vi "Simple 48-bit adder.vi"(8 "Input Valid":bool=TRUE, 10 "B":fxp<+/-,48,48>, 11 "A":fxp<+/-,48,48>) -> (0 "Output Valid":bool=TRUE, 3 "A+B":fxp<+/-,48,48>)   [LabVIEW 2012]
doc: "This VI adds two 48-bit numbers using DSP48E. The output is a 49-bit and carryout logic of DSP48E is used for this purpose."
uses:
  <vilib>/rvi/FXPMathLib/basic elements/DSP48E/simVIs/niFpgaDsp48eSimulationState.ctl
  <vilib>/rvi/FXPMathLib/basic elements/DSP48E/subVIs/niFpgaDsp48eType.ctl
  <vilib>/rvi/FXPMathLib/basic elements/DSP48E/subVIs/niFpgaDsp48eAlumodeOpmodeCarryinselState.ctl
  <vilib>/rvi/FXPMathLib/basic elements/DSP48E/subVIs/niFpgaDsp48eUseMultiplierState.ctl
  <vilib>/rvi/FXPMathLib/basic elements/DSP48E/subVIs/niFpgaDsp48eLogicUnitModeState.ctl
  <vilib>/rvi/FXPMathLib/basic elements/DSP48E/subVIs/niFpgaDsp48eSelectPatternState.ctl
  <vilib>/rvi/FXPMathLib/basic elements/DSP48E/subVIs/niFpgaDsp48eSelectMaskState.ctl
  <vilib>/rvi/FXPMathLib/basic elements/DSP48E/subVIs/niFpgaDsp48eAutoresetState.ctl
  <vilib>/rvi/FXPMathLib/basic elements/DSP48E/simVIs/niFpgaDsp48eResets.ctl
  <vilib>/rvi/FXPMathLib/basic elements/DSP48E/simVIs/niFpgaDsp48eEnables.ctl
  <vilib>/rvi/FXPMathLib/basic elements/DSP48E/simVIs/niFpgaDsp48eRegisters.ctl
  <vilib>/rvi/FXPMathLib/basic elements/DSP48E/simVIs/niFpgaDsp48eSimMultiplier.vi
  <vilib>/rvi/FXPMathLib/basic elements/DSP48E/simVIs/niFpgaDsp48eSimArithmetic.vi
  <vilib>/rvi/FXPMathLib/basic elements/DSP48E/simVIs/niFpgaDsp48eSimPatternDetect.vi
  <vilib>/rvi/FXPMathLib/basic elements/DSP48E/simVIs/niFpgaDsp48eSimP.vi
  <vilib>/rvi/FXPMathLib/basic elements/DSP48E/simVIs/niFpgaDsp48eSimUpdateState.vi
  <vilib>/rvi/FXPMathLib/basic elements/DSP48E/simVIs/niFpgaDsp48eCheckMode.vi
  <vilib>/rvi/FXPMathLib/basic elements/DSP48E/simVIs/niFpgaDsp48eReportInvalidMode.vi
  <vilib>/rvi/FXPMathLib/basic elements/FxpDiscreteDelay/XNode/nifxpmath_DiscreteDelay.xnode
  <vilib>/rvi/FXPMathLib/basic elements/DSP48E/XNode/niFpgaDsp48e.xnode
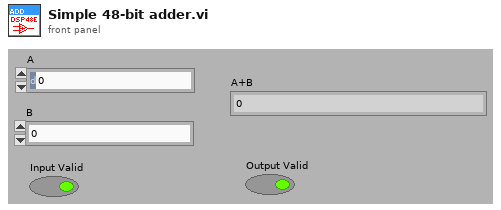
[diagram p1: front panel]
types:
  T1 = typedef "niFpgaDsp48eRegisters.ctl" = cluster{"a register 1":fxp<+/-,30,30>, "a register 2":fxp<+/-,30,30>, "b register 1":fxp<+/-,18,18>, "b register 2":fxp<+/-,18,18>, "c register":fxp<+/-,48,48>, "d register":fxp<+/-,25,25>, "ad register":fxp<+/-,25,25>, "m register":fxp<+/-,43,43>, "opmode register":fxp<+,7,7>, "alumode register":fxp<+,4,4>, "carryinsel register":fxp<+,3,3>, "inmode register":fxp<+,5,5>, "carryin register":bool, "multcarryin register":bool, "p registers":fxp<+/-,48,48>, "carryout register":fxp<+,4,4>, "carrycascout register":bool, "multsignout register":bool, "patterndetect register":bool, "patternbdetect register":bool, "patterndetect register 2":bool, "patternbdetect register 2":bool}
  T2 = typedef "niFpgaDsp48eEnables.ctl" = cluster{"cea1":bool, "cea2":bool, "cead":bool, "cealumode":bool, "ceb1":bool, "ceb2":bool, "cec":bool, "cecarryin":bool, "cectrl":bool, "ced":bool, "ceinmode":bool, "cem":bool, "cemultcarryin":bool, "cep":bool}
  T3 = typedef "niFpgaDsp48eResets.ctl" = cluster{"rsta":bool, "rstallcarryin":bool, "rstalumode":bool, "rstb":bool, "rstc":bool, "rstctrl":bool, "rstd":bool, "rstinmode":bool, "rstm":bool, "rstp":bool}
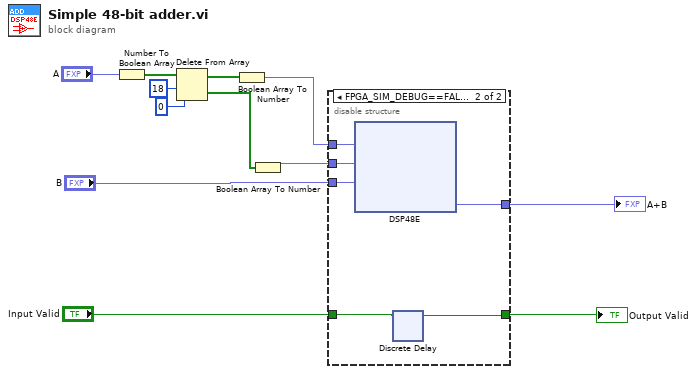
[diagram p0: block diagram]
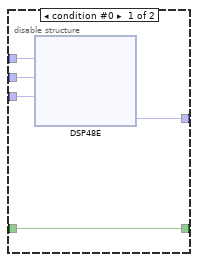
[diagram p2: hidden frame]
diagram:
  n1 = Number To Boolean Array(number="A") -> (Boolean array=w6:bool[])
  n2 = Delete From Array(array=w6, length=18, index=0) -> (deleted portion=w4:bool[], array with subset deleted=w5:bool[])
  n3 = Boolean Array To Number(Boolean array=w5) -> (number=w7:fxp<+/-,30,30>)
  n4 = Boolean Array To Number(Boolean array=w4) -> (number=w8:fxp<+/-,18,18>)
  n5 = disable-structure shown="FPGA_SIM_DEBUG==FALSE, default" {
    disable-tunnel: "B" -> [w17 w84]
    disable-tunnel: w8 -> [w16 w83]
    disable-tunnel: w7 -> [w15 w82]
    disable-tunnel: [w14 w81] -> w3
    disable-tunnel: "Input Valid" -> [w13 w80]
    disable-tunnel: [w13 w79] -> w1
    frame condition #0 {
      n6 = xnode "DSP48E"("a"=w15, "b"=w16, "c"=w17) -> ("p"=w14:fxp<+/-,48,48>)
    }
    frame condition #1 (active) {
      n7 = xnode "DSP48E"("a"=w82, "b"=w83, "c"=w84) -> ("p"=w81:fxp<+/-,48,48>)
      n8 = xnode "Discrete Delay"("D"=w80) -> ("Q"=w79:bool)
    }
  }
  "A+B" <- w3
  "Output Valid" <- w1
